vi "Begin.vi"() -> (0 "error out":errorcluster)   [LabVIEW 2011]
doc: "Called before other user functions, this VI is expected to open initial I/O refnums, load in file data, and do all program initialization. Notice that the <B>error out</B> terminal is simply used for data flow. Wiring it to other structures or subVIs ensures that this VI runs first."
uses:
  <vilib>/Rock Robotics/WPI/Joystick/WPI_JoystickDeviceEnum.ctl
  <vilib>/Rock Robotics/SystemInterfaces/DIO/FPGA_DIOChannel.ctl
  <vilib>/Rock Robotics/WPI/Encoder/WPI_EncoderType.ctl
  <vilib>/Rock Robotics/SystemInterfaces/Typedef/FPGA_TypedefAnalogModuleForGyro.ctl
  <vilib>/Rock Robotics/SystemInterfaces/AI/FPGA_AIGyroChannel.ctl
  <vilib>/Rock Robotics/SystemInterfaces/DIO/FPGA_DIOPWMChannel.ctl
  <vilib>/Rock Robotics/SystemInterfaces/DIO/FPGA_DIORelayChannel.ctl
  <vilib>/Rock Robotics/SystemInterfaces/Typedef/FPGA_TypedefSolenoidModule.ctl
  <vilib>/Rock Robotics/WPI/Solenoid/WPI_SolenoidChannel.ctl
  <vilib>/Rock Robotics/WPI/Solenoid/WPI_SolenoidValue.ctl
  <vilib>/Rock Robotics/WPI/Camera/WPI_CameraWhite Balance Values.ctl
  <vilib>/Rock Robotics/WPI/Camera/WPI_CameraExposure Values.ctl
  <vilib>/Rock Robotics/WPI/Camera/WPI_CameraFrameRate.ctl
  <vilib>/Rock Robotics/WPI/Camera/WPI_CameraImageSize.ctl
  <vilib>/Rock Robotics/SystemInterfaces/Typedef/FPGA_TypedefDigitalModule.ctl
  ADXL345 I2C Range.ctl
  <vilib>/Rock Robotics/WPI/Counter/WPI_CounterDigitalInputToDigitalSource.vi
  <vilib>/Rock Robotics/WPI/MotorControl/WPI_MotorControlOpen Jaguar.vi
  <vilib>/Rock Robotics/WPI/RobotDrive/WPI_RobotDriveOpen4MotorWithJaguar.vi
  <vilib>/Rock Robotics/WPI/Solenoid/WPI_SolenoidOpenDouble.vi
  <vilib>/Rock Robotics/WPI/Solenoid/WPI_SolenoidSetEnum.vi
  <vilib>/Rock Robotics/WPI/Compressor/WPI_CompressorGetSetRefNum.vi
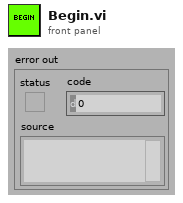
[diagram p1: front panel]
types:
  T1 = typedef "ADXL345 I2C Range.ctl" = u8
  T2 = typedef "FPGA_TypedefDigitalModule.ctl" = enum16{"Digital Module 1", "Digital Module 2"}
  T3 = typedef "FPGA_DIOChannel.ctl" = enum8{"DIO 1", "DIO 2", "DIO 3", "DIO 4", "DIO 5", "DIO 6", "DIO 7", "DIO 8", "DIO 9", "DIO 10", "DIO 11", "DIO 12", "DIO 13", "DIO 14", "Invalid"}
  T4 = typedef "WPI_SolenoidValue.ctl" = enum16{"Off", "On", "Forward", "Reverse"}
  T5 = typedef "WPI_SolenoidChannel.ctl" = enum8{"Solenoid 1", "Solenoid 2", "Solenoid 3", "Solenoid 4", "Solenoid 5", "Solenoid 6", "Solenoid 7", "Solenoid 8", "Invalid"}
  T6 = typedef "FPGA_TypedefSolenoidModule.ctl" = enum16{"Solenoid Module 1", "Solenoid Module 2"}
  T7 = typedef "WPI_CameraImageSize.ctl" = enum16{"640x480", "320x240", "160x120"}
  T8 = typedef "WPI_CameraFrameRate.ctl" = u32
  T9 = typedef "WPI_CameraExposure Values.ctl" = enum16{"Auto", "Flicker-free 50 Hz", "Flicker-free 60 Hz", "Hold current"}
  T10 = typedef "WPI_CameraWhite Balance Values.ctl" = enum16{"Auto", "Fixed indoor", "Fixed outdoor 1", "Fixed outdoor 2", "Fixed fluorescent 1", "Fixed fluorescent 2", "Hold current"}
  T11 = typedef "FPGA_DIORelayChannel.ctl" = enum8{"Relay 1", "Relay 2", "Relay 3", "Relay 4", "Relay 5", "Relay 6", "Relay 7", "Relay 8", "Invalid"}
  T12 = typedef "FPGA_DIOPWMChannel.ctl" = enum8{"PWM 1", "PWM 2", "PWM 3", "PWM 4", "PWM 5", "PWM 6", "PWM 7", "PWM 8", "PWM 9", "PWM 10", "Invalid"}
  T13 = typedef "FPGA_AIGyroChannel.ctl" = enum8{"AI 1", "AI 2", "Invalid"}
  T14 = typedef "FPGA_TypedefAnalogModuleForGyro.ctl" = enum16{"Analog Module 1"}
  T15 = typedef "WPI_EncoderType.ctl" = enum16{"1x", "2x", "4x"}
  T16 = typedef "WPI_JoystickDeviceEnum.ctl" = enum16{"USB 1", "USB 2", "USB 3", "USB 4", "Kinect 1", "Kinect 2"}
  T17 = typedef "WPI_JoystickDevRef.ctl" = cluster{"Device":T16}
  T18 = typedef "WPI_CompressorDevRef.ctl" = cluster{"DevStatus":errorcluster, "DigitalInputDevRef":T19, "RelayDevRef":T20}
  T19 = typedef "WPI_DigitalInputDevRef.ctl" = cluster{"DevStatus":errorcluster, "DIO Channel":T3, "Digital Module":T2}
  T20 = typedef "WPI_RelayDevRef.ctl" = cluster{"DevStatus":errorcluster, "Relay Channel":T11, "Digital Module":T2, "Relay Direction":T21}
  T21 = typedef "WPI_RelayDirection.ctl" = enum16{"Both directions", "Forward only", "Reverse only"}
  T22 = typedef "WPI_MotorControlDeviceRef.ctl" = cluster{"DeviceStatus":errorcluster, "Type":enum16{"PWM", "CAN"}, "PWM":cluster{"Digital Module":T2, "PWM Channel":T12, "DeadBand":T23}, "CAN":cluster{"Device Number":u8, "Control Mode":T24, "Semaphore":T25, "Max Vout":dbl}, "Invert":bool, "TransformRef":T26, "InvTransformRef":T26}
  T23 = typedef "WPI_PWMDeadband.ctl" = cluster{"Name":string, "maxPositivePwm":i32, "minPositivePwm":i32, "centerPwm":i32, "maxNegativePwm":i32, "minNegativePwm":i32, "angularRange":u16}
  T24 = typedef "WPI_CANJaguar_ControlMode.ctl" = enum8{"Percent VBus", "Current", "Speed", "Position", "Voltage"}
  T25 = typedef "Semaphore RefNum" = refnum<k1>
  T26 = typedef "WPI_PWMTransform_ConPane.ctl" = refnum<vi>
  T27 = typedef "WPI_SolenoidDevRef.ctl" = cluster{"DevStatus":errorcluster, "Solenoid Module":T6, "Forward Solenoid Channel":T5, "Reverse Solenoid Channel":T5}
  T28 = typedef "WPI_CameraDevRef.ctl" = cluster{"Camera Address":string, "CameraStatus":errorcluster, "Acquire Image Notifier":refnum<notifier>}
  T29 = typedef "FPGA_CounterEncoderSourceConvertionLVSourceType.ctl" = cluster{"DevStatus":errorcluster, "AnalogTriggerMode?":bool, "DigitalMode":cluster{"Digital Module":T2, "DIO Channel":T30}, "AnalogTriggerMode":cluster{"AnalogTriggerIndex":T31, "OutputType":T32}}
  T30 = typedef "FPGA_DIODigitalSourceChannel.ctl" = enum8{"DIO 1", "DIO 2", "DIO 3", "DIO 4", "DIO 5", "DIO 6", "DIO 7", "DIO 8", "DIO 9", "DIO 10", "DIO 11", "DIO 12", "DIO 13", "DIO 14", "Disabled"}
  T31 = typedef "FPGA_AnalogTriggerIndex.ctl" = enum8{"Trig 0", "Trig 1", "Trig 2", "Trig 3", "Trig 4", "Trig 5", "Trig 6", "Trig 7", "Invalid"}
  T32 = typedef "FPGA_AnalogTriggerOutType.ctl" = enum16{"InWindow", "TriggerState", "Rising", "Falling"}
  T33 = typedef "WPI_RobotDriveDevRef.ctl" = cluster{"DevStatus":errorcluster, "Motors[]":T22[], "Square Inputs":bool, "Max Output":dbl, "Isochronous":bool}
  T34 = typedef "WPI_GyroDevRef.ctl" = cluster{"DevStatus":errorcluster, "Analog Module":T35, "Analog Channel":T36, "Offset":dbl, "Gain (VoltsPerDegree/Second)":dbl}
  T35 = typedef "FPGA_TypedefAnalogModule.ctl" = enum16{"Analog Module 1", "Analog Module 2"}
  T36 = typedef "FPGA_AIChannel.ctl" = enum8{"AI 1", "AI 2", "AI 3", "AI 4", "AI 5", "AI 6", "AI 7", "AI 8", "Invalid"}
  T37 = typedef "WPI_I2CDevRef.ctl" = cluster{"DevStatus":errorcluster, "Digital Module":T2, "Device Address":u8}
  T38 = typedef "WPI_EncoderDevRef.ctl" = cluster{"DevStatus":errorcluster, "EncoderIndex":T39, "CounterIndex":T40, "DistancePerCount":dbl, "Decoding Type":T15}
  T39 = typedef "FPGA_EncoderIdx.ctl" = enum8{"Enc 0", "Enc 1", "Enc 2", "Enc 3", "Invalid"}
  T40 = typedef "FPGA_CounterCtrSystemIndex.ctl" = enum8{"Ctr 0", "Ctr 1", "Ctr 2", "Ctr 3", "Ctr 4", "Ctr 5", "Ctr 6", "Ctr 7", "Invalid"}
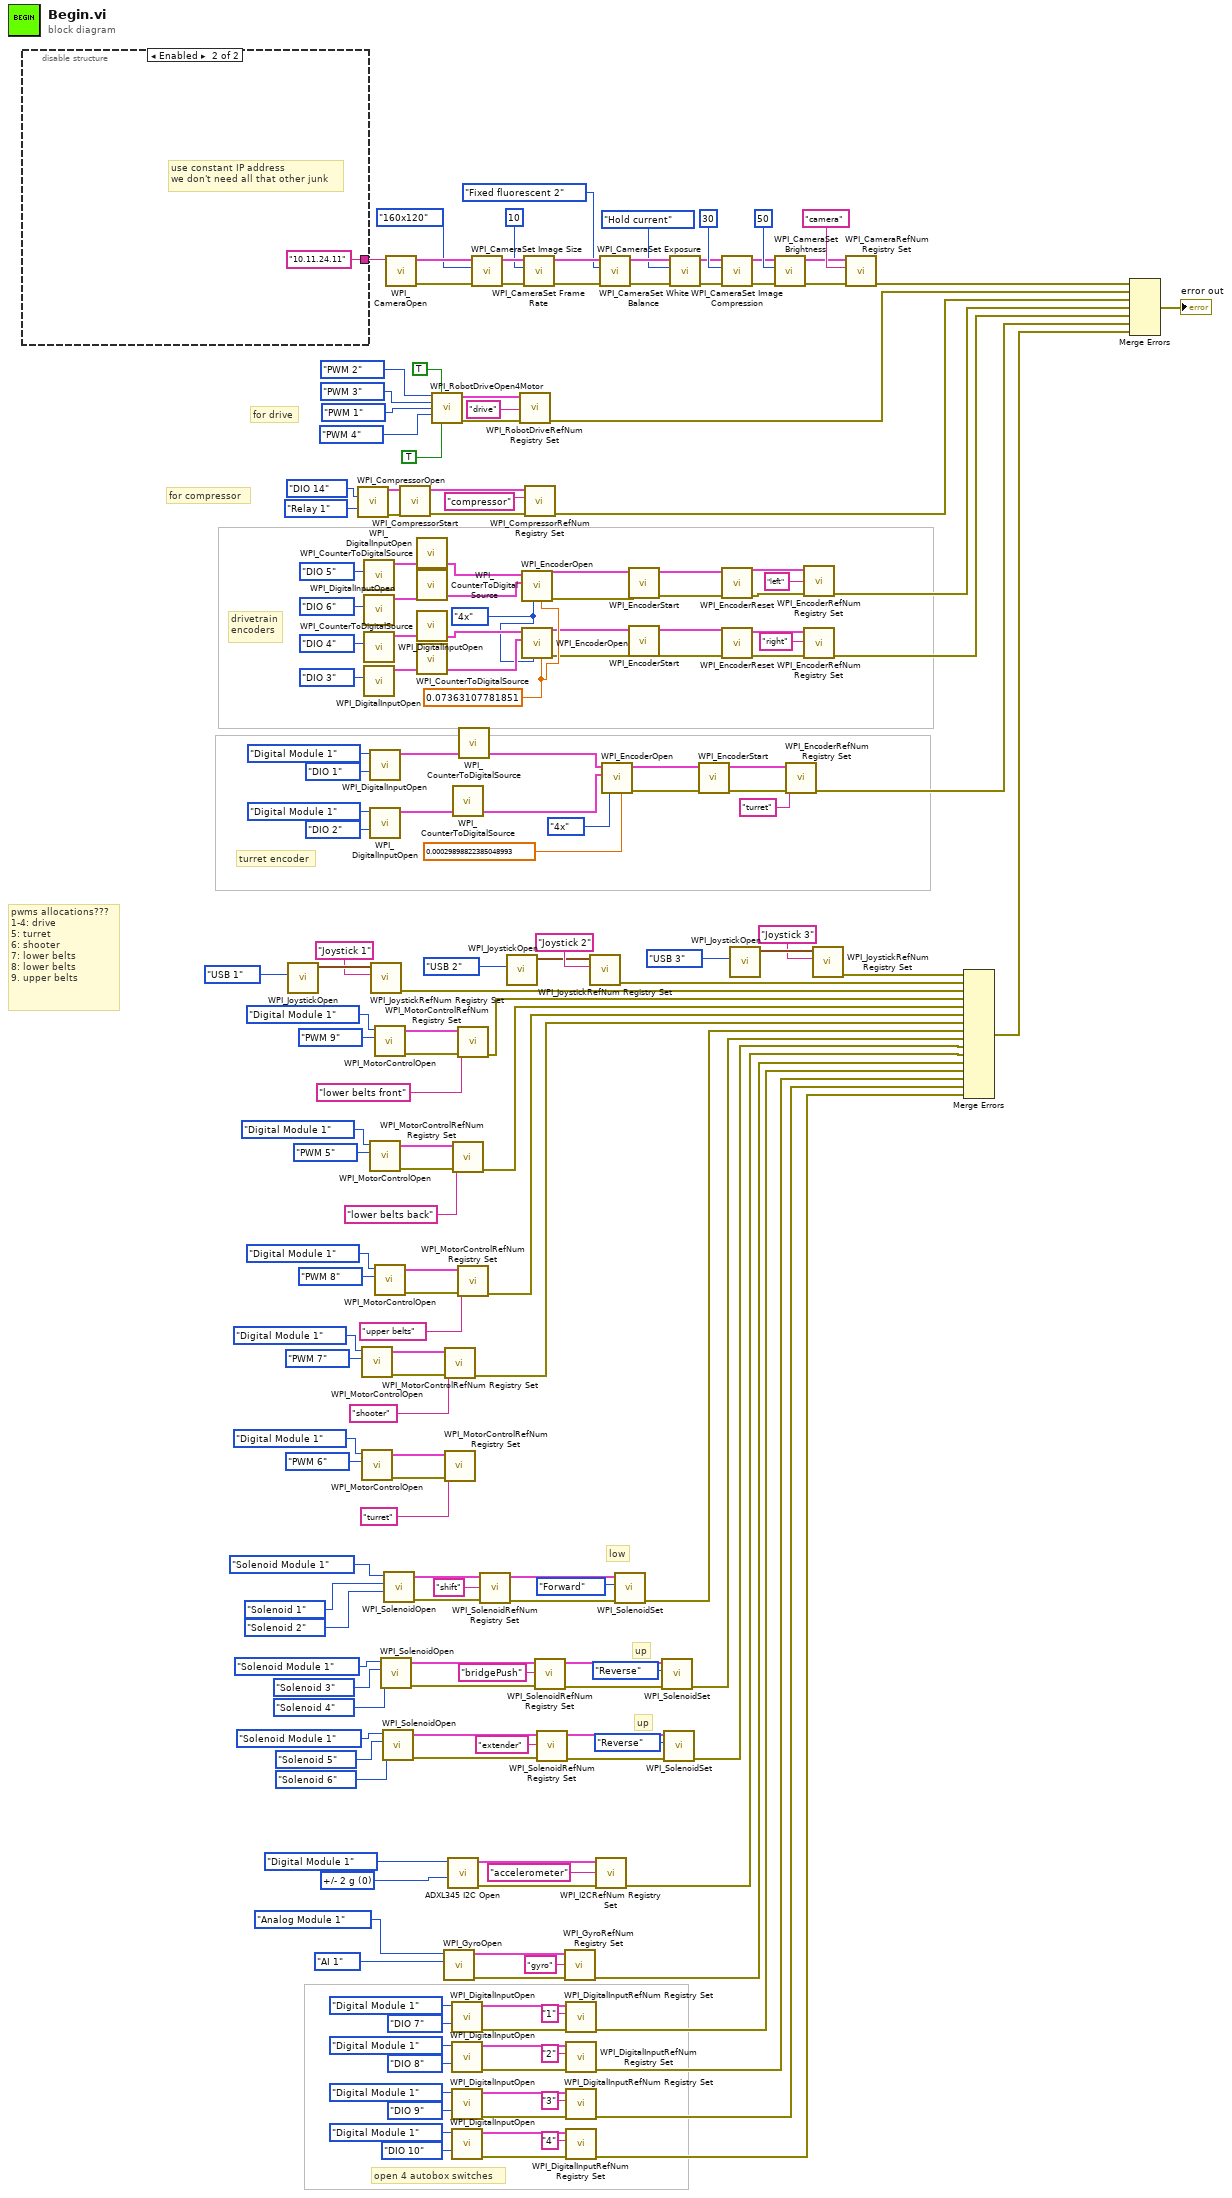
[diagram p0: block diagram]
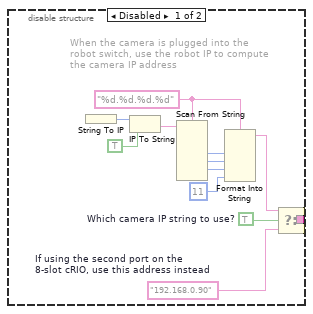
[diagram p2: hidden frame]
diagram:
  w6 = T1 0 items=["+/- 2 g", "+/- 4 g", "+/- 8 g", "+/- 16 g"] ("Range")
  w146 = 0.07363107781851 ("DistancePerCount")
  w147 = WPI_EncoderType."4x" ("Decoding Type")
  # "open 4 autobox switches"
  # "up"
  # "up"
  # "low"
  # "pwms allocations???\n1-4: drive\n5: turret\n6: shooter\n7: lower belts\n8: lower belts\n9. upper belts"
  # "turret encoder"
  # "for compressor"
  # "for drive"
  # "drivetrain\nencoders"
  n1 = disable-structure shown="Enabled" {
    disable-tunnel: [w200 "10.11.24.11" ("Camera Address")] -> w193
    frame Disabled {
      w197 = TRUE  # Which camera IP string to use?
      w201 = "%d.%d.%d.%d" ("format string")
      w198 = "192.168.0.90"  # If using the second port on the 8-slot cRIO, use this address instead
      # "When the camera is plugged into the\nrobot switch, use the robot IP to compute\nthe camera IP address"
      n2 = String To IP() -> (0:w208:u32)  [unwired: 1 in]
      n3 = IP To String(1:TRUE ("dot notation? (F)"), 2:w208) -> (0:w206:string)
      n4 = Scan From String(format string=w201, input string=w206) -> (output 1=w205:i32, output 2=w204:i32, output 3=w203:i32)  [unwired: 7 in, 3 out]
      n5 = Format Into String(format string=w201, w205, w204, w203, 11 ("Compression")) -> (resulting string=w199:string)  [unwired: 2 in, 1 out]
      n6 = Select(t=w199, s=w197, f=w198) -> (s? t:f=w200:string)
    }
    frame Enabled {
      # "use constant IP address\nwe don't need all that other junk"
    }
  }
  n7 = call <vilib>:"WPI_JoystickOpen.vi"("JoystickDevice"=WPI_JoystickDeviceEnum."USB 1") -> ("JoystickDevRef"=w196:T17)  [unwired: 10 out]
  n8 = call <vilib>:"WPI_CompressorOpen.vi"("Pressure Switch DIO Channel"=FPGA_DIOChannel."DIO 14", "Relay Channel"=FPGA_DIORelayChannel."Relay 1") -> ("CompressorDevRef"=w90:T18, "error out"=w89:errorcluster)  [unwired: 12 in]
  n9 = call-poly <vilib>:"WPI_MotorControlOpen.vi"("PWM Channel"=FPGA_DIOPWMChannel."PWM 7", "Digital Module (Module 1)"=FPGA_TypedefDigitalModule."Digital Module 1") -> ("error out"=w109:errorcluster, "MotorControlDeviceRef"=w108:T22)  [unwired: 8 in]
  n10 = call-poly <vilib>:"WPI_MotorControlOpen.vi"("PWM Channel"=FPGA_DIOPWMChannel."PWM 6", "Digital Module (Module 1)"=FPGA_TypedefDigitalModule."Digital Module 1") -> ("error out"=w114:errorcluster, "MotorControlDeviceRef"=w115:T22)  [unwired: 8 in]
  n11 = call <vilib>:"WPI_DigitalInputOpen.vi"("DIO Channel"=FPGA_DIOChannel."DIO 5") -> ("DigitalInputDevRef"=w64:T19)  [unwired: 9 in, 1 out]
  n12 = call <vilib>:"WPI_DigitalInputOpen.vi"("DIO Channel"=FPGA_DIOChannel."DIO 6") -> ("DigitalInputDevRef"=w63:T19)  [unwired: 9 in, 1 out]
  n13 = call <vilib>:"WPI_DigitalInputOpen.vi"("DIO Channel"=FPGA_DIOChannel."DIO 4") -> ("DigitalInputDevRef"=w68:T19)  [unwired: 9 in, 1 out]
  n14 = call <vilib>:"WPI_DigitalInputOpen.vi"("DIO Channel"=FPGA_DIOChannel."DIO 3") -> ("DigitalInputDevRef"=w67:T19)  [unwired: 9 in, 1 out]
  n15 = call <vilib>:"WPI_DigitalInputOpen.vi"("DIO Channel"=FPGA_DIOChannel."DIO 1", "Digital Module (Module 1)"=FPGA_TypedefDigitalModule."Digital Module 1") -> ("DigitalInputDevRef"=w188:T19)  [unwired: 8 in, 1 out]
  n16 = call <vilib>:"WPI_DigitalInputOpen.vi"("DIO Channel"=FPGA_DIOChannel."DIO 2", "Digital Module (Module 1)"=FPGA_TypedefDigitalModule."Digital Module 1") -> ("DigitalInputDevRef"=w187:T19)  [unwired: 8 in, 1 out]
  n17 = call-poly <vilib>:"WPI_MotorControlOpen.vi"("PWM Channel"=FPGA_DIOPWMChannel."PWM 5", "Digital Module (Module 1)"=FPGA_TypedefDigitalModule."Digital Module 1") -> ("error out"=w104:errorcluster, "MotorControlDeviceRef"=w103:T22)  [unwired: 8 in]
  n18 = call <vilib>:"WPI_JoystickRefNum Registry Set.vi"("refnum name"="Joystick 1", "JoystickDevRef"=w196) -> ("error out"=w161:errorcluster)  [unwired: 1 in, 8 out]
  n19 = call-poly <vilib>:"WPI_MotorControlOpen.vi"("PWM Channel"=FPGA_DIOPWMChannel."PWM 9", "Digital Module (Module 1)"=FPGA_TypedefDigitalModule."Digital Module 1") -> ("error out"=w124:errorcluster, "MotorControlDeviceRef"=w125:T22)  [unwired: 8 in]
  n20 = call-poly <vilib>:"WPI_MotorControlOpen.vi"("PWM Channel"=FPGA_DIOPWMChannel."PWM 8", "Digital Module (Module 1)"=FPGA_TypedefDigitalModule."Digital Module 1") -> ("error out"=w119:errorcluster, "MotorControlDeviceRef"=w118:T22)  [unwired: 8 in]
  n21 = call-poly <vilib>:"WPI_SolenoidOpen.vi"("Reverse Solenoid Channel"=WPI_SolenoidChannel."Solenoid 4", "Forward Solenoid Channel"=WPI_SolenoidChannel."Solenoid 3" ("Solenoid Channel"), "Solenoid Module (Module 1)"=FPGA_TypedefSolenoidModule."Solenoid Module 1") -> ("error out"=w74:errorcluster, "SolenoidDevRef"=w73:T27)  [unwired: 7 in]
  n22 = call-poly <vilib>:"WPI_SolenoidOpen.vi"("Reverse Solenoid Channel"=WPI_SolenoidChannel."Solenoid 6", "Forward Solenoid Channel"=WPI_SolenoidChannel."Solenoid 5" ("Solenoid Channel"), "Solenoid Module (Module 1)"=FPGA_TypedefSolenoidModule."Solenoid Module 1") -> ("error out"=w36:errorcluster, "SolenoidDevRef"=w37:T27)  [unwired: 7 in]
  n23 = call-poly <vilib>:"WPI_SolenoidOpen.vi"("Reverse Solenoid Channel"=WPI_SolenoidChannel."Solenoid 2", "Forward Solenoid Channel"=WPI_SolenoidChannel."Solenoid 1" ("Solenoid Channel"), "Solenoid Module (Module 1)"=FPGA_TypedefSolenoidModule."Solenoid Module 1") -> ("error out"=w81:errorcluster, "SolenoidDevRef"=w82:T27)  [unwired: 7 in]
  n24 = call <vilib>:"WPI_CameraOpen.vi"("Camera Address"=w193) -> ("error out"=w53:errorcluster, "CameraDevRef"=w54:T28)  [unwired: 1 in, 8 out]
  n25 = call <vilib>:"WPI_CompressorStart.vi"("error in (no error)"=w89, "CompressorDevRef"=w90) -> ("error out"=w87:errorcluster, "CompressorDevRef"=w88:T18)  [unwired: 8 in]
  n26 = call-poly <vilib>:"WPI_CounterToDigitalSource.vi"("DigitalInputDevRef"=w64) -> ("Digital Source"=w151:T29)  [unwired: 6 in]
  n27 = call-poly <vilib>:"WPI_CounterToDigitalSource.vi"("DigitalInputDevRef"=w63) -> ("Digital Source"=w150:T29)  [unwired: 6 in]
  n28 = call-poly <vilib>:"WPI_CounterToDigitalSource.vi"("DigitalInputDevRef"=w68) -> ("Digital Source"=w149:T29)  [unwired: 6 in]
  n29 = call-poly <vilib>:"WPI_CounterToDigitalSource.vi"("DigitalInputDevRef"=w67) -> ("Digital Source"=w148:T29)  [unwired: 6 in]
  n30 = call-poly <vilib>:"WPI_RobotDriveOpen4Motor.vi"("Rear Left Motor"=FPGA_DIOPWMChannel."PWM 2", "Rear Left Motor Inverted"=TRUE ("Rear Right Motor Inverted"), "Rear Right Motor"=FPGA_DIOPWMChannel."PWM 3", "Front Left Motor"=FPGA_DIOPWMChannel."PWM 1", "Front Right Motor"=FPGA_DIOPWMChannel."PWM 4", "Front Left Motor Inverted"=TRUE ("Front Right Motor Inverted")) -> ("RobotDriveDevRef"=w97:T33, "error out"=w96:errorcluster)  [unwired: 8 in]
  n31 = call <vilib>:"WPI_GyroOpen.vi"("Analog Channel"=FPGA_AIGyroChannel."AI 1", "Analog Module (Module 1)"=FPGA_TypedefAnalogModuleForGyro."Analog Module 1") -> ("error out"=w129:errorcluster, "GyroDevRef"=w128:T34)  [unwired: 7 in, 1 out]
  n32 = call <vilib>:"WPI_MotorControlRefNum Registry Set.vi"("error in (no error)"=w109, "refnum name"="shooter", "MotorControlDevRef"=w108) -> ("error out"=w157:errorcluster)  [unwired: 7 in, 1 out]
  n33 = call <vilib>:"WPI_MotorControlRefNum Registry Set.vi"("error in (no error)"=w114, "refnum name"="turret", "MotorControlDevRef"=w115) -> ()  [unwired: 7 in, 2 out]
  n34 = call "ADXL345 I2C Open.vi"("Range"=w6, "DIO Module (Slot 4)"=FPGA_TypedefDigitalModule."Digital Module 1" ("DIO Module")) -> ("error out"=w8:errorcluster, "I2CDevRef"=w9:T37)  [unwired: 2 in, 6 out]
  n35 = call <vilib>:"WPI_DigitalInputOpen.vi"("DIO Channel"=FPGA_DIOChannel."DIO 7", "Digital Module (Module 1)"=FPGA_TypedefDigitalModule."Digital Module 1") -> ("error out"=w27:errorcluster, "DigitalInputDevRef"=w26:T19)  [unwired: 8 in]
  n36 = call <vilib>:"WPI_DigitalInputOpen.vi"("DIO Channel"=FPGA_DIOChannel."DIO 8", "Digital Module (Module 1)"=FPGA_TypedefDigitalModule."Digital Module 1") -> ("error out"=w24:errorcluster, "DigitalInputDevRef"=w25:T19)  [unwired: 8 in]
  n37 = call <vilib>:"WPI_DigitalInputOpen.vi"("DIO Channel"=FPGA_DIOChannel."DIO 9", "Digital Module (Module 1)"=FPGA_TypedefDigitalModule."Digital Module 1") -> ("error out"=w16:errorcluster, "DigitalInputDevRef"=w17:T19)  [unwired: 8 in]
  n38 = call <vilib>:"WPI_DigitalInputOpen.vi"("DIO Channel"=FPGA_DIOChannel."DIO 10", "Digital Module (Module 1)"=FPGA_TypedefDigitalModule."Digital Module 1") -> ("error out"=w19:errorcluster, "DigitalInputDevRef"=w18:T19)  [unwired: 8 in]
  n39 = call-poly <vilib>:"WPI_CounterToDigitalSource.vi"("DigitalInputDevRef"=w187) -> ("Digital Source"=w185:T29)  [unwired: 6 in]
  n40 = call <vilib>:"WPI_MotorControlRefNum Registry Set.vi"("error in (no error)"=w104, "refnum name"="lower belts back", "MotorControlDevRef"=w103) -> ("error out"=w159:errorcluster)  [unwired: 7 in, 1 out]
  n41 = call <vilib>:"WPI_MotorControlRefNum Registry Set.vi"("error in (no error)"=w124, "refnum name"="lower belts front", "MotorControlDevRef"=w125) -> ("error out"=w160:errorcluster)  [unwired: 7 in, 1 out]
  n42 = call <vilib>:"WPI_MotorControlRefNum Registry Set.vi"("error in (no error)"=w119, "refnum name"="upper belts", "MotorControlDevRef"=w118) -> ("error out"=w158:errorcluster)  [unwired: 7 in, 1 out]
  n43 = call-poly <vilib>:"WPI_CounterToDigitalSource.vi"("DigitalInputDevRef"=w188) -> ("Digital Source"=w186:T29)  [unwired: 6 in]
  n44 = call <vilib>:"WPI_CameraSet Image Size.vi"("error in (no error)"=w53, "Image Size"=WPI_CameraImageSize."160x120", "CameraDevRef"=w54) -> ("error out"=w52:errorcluster, "CameraDevRef Out"=w55:T28)  [unwired: 7 out]
  n45 = call <vilib>:"WPI_SolenoidRefNum Registry Set.vi"("error in (no error)"=w81, "refnum name"="shift", "SolenoidDevRef"=w82) -> ("error out"=w78:errorcluster, "SolenoidDevRef"=w79:T27)  [unwired: 7 in]
  n46 = call <vilib>:"WPI_JoystickOpen.vi"("JoystickDevice"=WPI_JoystickDeviceEnum."USB 2") -> ("JoystickDevRef"=w175:T17)  [unwired: 10 out]
  n47 = call <vilib>:"WPI_RobotDriveRefNum Registry Set.vi"("error in (no error)"=w96, "refnum name"="drive", "RobotDriveDevRef"=w97) -> ("error out"=w169:errorcluster)  [unwired: 7 in, 1 out]
  n48 = call <vilib>:"WPI_EncoderOpen.vi"("DistancePerCount"=w146, "Decoding Type"=w147, "BSource"=w150, "ASource"=w151) -> ("error out"=w138:errorcluster, "EncoderDevRef"=w139:T38)  [unwired: 6 in]
  n49 = call <vilib>:"WPI_EncoderOpen.vi"("DistancePerCount"=w146, "Decoding Type"=w147, "BSource"=w148, "ASource"=w149) -> ("error out"=w134:errorcluster, "EncoderDevRef"=w135:T38)  [unwired: 6 in]
  n50 = call <vilib>:"WPI_CameraSet Frame Rate.vi"("error in (no error)"=w52, "Frame Rate (fps)"=T8 10, "CameraDevRef"=w55) -> ("error out"=w51:errorcluster, "CameraDevRef Out"=w57:T28)  [unwired: 7 out]
  n51 = call <vilib>:"WPI_CompressorRefNum Registry Set.vi"("error in (no error)"=w87, "refnum name"="compressor", "CompressorDevRef"=w88) -> ("error out"=w168:errorcluster)  [unwired: 7 in, 1 out]
  n52 = call <vilib>:"WPI_SolenoidRefNum Registry Set.vi"("error in (no error)"=w74, "refnum name"="bridgePush", "SolenoidDevRef"=w73) -> ("error out"=w77:errorcluster, "SolenoidDevRef"=w76:T27)  [unwired: 7 in]
  n53 = call <vilib>:"WPI_SolenoidRefNum Registry Set.vi"("error in (no error)"=w36, "refnum name"="extender", "SolenoidDevRef"=w37) -> ("error out"=w33:errorcluster, "SolenoidDevRef"=w34:T27)  [unwired: 7 in]
  n54 = call <vilib>:"WPI_GyroRefNum Registry Set.vi"("error in (no error)"=w129, "refnum name"="gyro", "GyroDevRef"=w128) -> ("error out"=w32:errorcluster)  [unwired: 7 in, 1 out]
  n55 = call <vilib>:"WPI_DigitalInputRefNum Registry Set.vi"("error in (no error)"=w27, "refnum name"="1", "DigitalInputDevRef"=w26) -> ("error out"=w4:errorcluster)  [unwired: 7 in, 1 out]
  n56 = call <vilib>:"WPI_DigitalInputRefNum Registry Set.vi"("error in (no error)"=w24, "refnum name"="2", "DigitalInputDevRef"=w25) -> ("error out"=w3:errorcluster)  [unwired: 7 in, 1 out]
  n57 = call <vilib>:"WPI_DigitalInputRefNum Registry Set.vi"("error in (no error)"=w16, "refnum name"="3", "DigitalInputDevRef"=w17) -> ("error out"=w2:errorcluster)  [unwired: 7 in, 1 out]
  n58 = call <vilib>:"WPI_DigitalInputRefNum Registry Set.vi"("error in (no error)"=w19, "refnum name"="4", "DigitalInputDevRef"=w18) -> ("error out"=w1:errorcluster)  [unwired: 7 in, 1 out]
  n59 = call <vilib>:"WPI_JoystickRefNum Registry Set.vi"("refnum name"="Joystick 2", "JoystickDevRef"=w175) -> ("error out"=w162:errorcluster)  [unwired: 1 in, 8 out]
  n60 = call <vilib>:"WPI_I2CRefNum Registry Set.vi"("error in (no error)"=w8, "refnum name"="accelerometer", "I2CDevRef"=w9) -> ("error out"=w31:errorcluster)  [unwired: 7 in, 1 out]
  n61 = call <vilib>:"WPI_CameraSet White Balance.vi"("error in (no error)"=w51, "White Balance"=WPI_CameraWhite_Balance_Values."Fixed fluorescent 2", "CameraDevRef"=w57) -> ("error out"=w50:errorcluster, "CameraDevRef Out"=w56:T28)  [unwired: 7 out]
  n62 = call <vilib>:"WPI_EncoderOpen.vi"("DistancePerCount"=0.00029898822385048993, "Decoding Type"=WPI_EncoderType."4x", "BSource"=w185, "ASource"=w186) -> ("error out"=w182:errorcluster, "EncoderDevRef"=w183:T38)  [unwired: 6 in]
  n63 = call-poly <vilib>:"WPI_SolenoidSet.vi"("error in (no error)"=w78, "Value"=WPI_SolenoidValue."Forward", "SolenoidDevRef"=w79) -> ("error out"=w156:errorcluster)  [unwired: 7 in, 1 out]
  n64 = call <vilib>:"WPI_EncoderStart.vi"("error in (no error)"=w138, "EncoderDevRef"=w139) -> ("error out"=w136:errorcluster, "EncoderDevRef"=w137:T38)  [unwired: 8 in]
  n65 = call <vilib>:"WPI_EncoderStart.vi"("error in (no error)"=w134, "EncoderDevRef"=w135) -> ("error out"=w132:errorcluster, "EncoderDevRef"=w133:T38)  [unwired: 8 in]
  n66 = call-poly <vilib>:"WPI_SolenoidSet.vi"("error in (no error)"=w77, "Value"=WPI_SolenoidValue."Reverse", "SolenoidDevRef"=w76) -> ("error out"=w85:errorcluster)  [unwired: 7 in, 1 out]
  n67 = call-poly <vilib>:"WPI_SolenoidSet.vi"("error in (no error)"=w33, "Value"=WPI_SolenoidValue."Reverse", "SolenoidDevRef"=w34) -> ("error out"=w30:errorcluster)  [unwired: 7 in, 1 out]
  n68 = call <vilib>:"WPI_CameraSet Exposure.vi"("error in (no error)"=w50, "Exposure"=WPI_CameraExposure_Values."Hold current", "CameraDevRef"=w56) -> ("error out"=w49:errorcluster, "CameraDevRef Out"=w59:T28)  [unwired: 7 out]
  n69 = call <vilib>:"WPI_EncoderStart.vi"("error in (no error)"=w182, "EncoderDevRef"=w183) -> ("error out"=w180:errorcluster, "EncoderDevRef"=w181:T38)  [unwired: 8 in]
  n70 = call <vilib>:"WPI_CameraSet Image Compression.vi"("error in (no error)"=w49, "Compression"=30, "CameraDevRef"=w59) -> ("error out"=w48:errorcluster, "CameraDevRef Out"=w58:T28)  [unwired: 7 out]
  n71 = call <vilib>:"WPI_EncoderReset.vi"("error in (no error)"=w136, "EncoderDevRef"=w137) -> ("error out"=w144:errorcluster, "EncoderDevRef"=w145:T38)  [unwired: 8 in]
  n72 = call <vilib>:"WPI_EncoderReset.vi"("error in (no error)"=w132, "EncoderDevRef"=w133) -> ("error out"=w143:errorcluster, "EncoderDevRef"=w142:T38)  [unwired: 8 in]
  n73 = call <vilib>:"WPI_JoystickOpen.vi"("JoystickDevice"=WPI_JoystickDeviceEnum."USB 3") -> ("JoystickDevRef"=w174:T17)  [unwired: 10 out]
  n74 = call <vilib>:"WPI_CameraSet Brightness.vi"("error in (no error)"=w48, "Brightness"=50, "CameraDevRef"=w58) -> ("error out"=w42:errorcluster, "CameraDevRef Out"=w43:T28)  [unwired: 7 out]
  n75 = call <vilib>:"WPI_EncoderRefNum Registry Set.vi"("error in (no error)"=w180, "refnum name"="turret", "EncoderDevRef"=w181) -> ("error out"=w165:errorcluster)  [unwired: 7 in, 1 out]
  n76 = call <vilib>:"WPI_EncoderRefNum Registry Set.vi"("error in (no error)"=w144, "refnum name"="left", "EncoderDevRef"=w145) -> ("error out"=w167:errorcluster)  [unwired: 7 in, 1 out]
  n77 = call <vilib>:"WPI_EncoderRefNum Registry Set.vi"("error in (no error)"=w143, "refnum name"="right", "EncoderDevRef"=w142) -> ("error out"=w166:errorcluster)  [unwired: 7 in, 1 out]
  n78 = call <vilib>:"WPI_JoystickRefNum Registry Set.vi"("refnum name"="Joystick 3", "JoystickDevRef"=w174) -> ("error out"=w163:errorcluster)  [unwired: 1 in, 8 out]
  n79 = call <vilib>:"WPI_CameraRefNum Registry Set.vi"("error in (no error)"=w42, "refnum name"="camera", "CameraDevRef"=w43) -> ("error out"=w170:errorcluster)  [unwired: 8 out]
  n80 = Merge Errors(w163, w162, w161, w160, w159, w158, w157, w156, w85, w30, w31, w32, w4, w3, w2, w1) -> (w164:errorcluster)
  n81 = Merge Errors(w170, w169, w168, w167, w166, w165, w164) -> (→"error out":errorcluster)
